vi "Read Plot Area Bounds.vi"(8 "error in (no error)":errorcluster, 11 "GraphChart.lvclass in":refnum<class "GraphChart.lvclass">) -> (0 "error out":errorcluster, 2 "Plot Bounds":T1, 3 "GraphChart.lvclass out":refnum<class "GraphChart.lvclass">)   [LabVIEW 2015, in "GraphChart.lvclass"]
uses:
  GraphChart.lvclass
  <vilib>/Utility/miscctls.llb/LVRectTypeDef.ctl
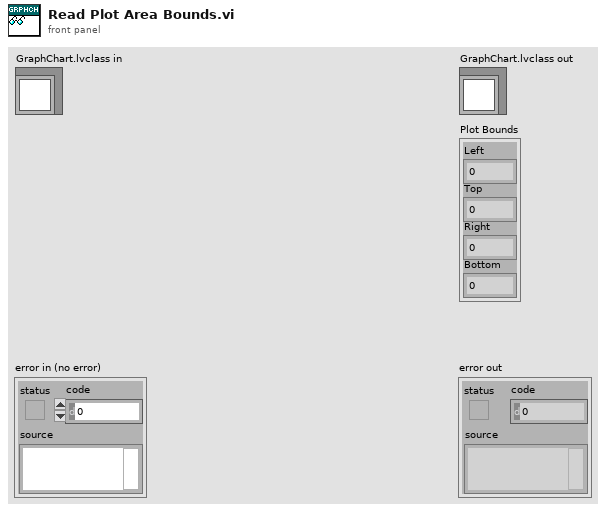
[diagram p1: front panel]
types:
  T1 = typedef "LVRectTypeDef.ctl" = cluster{"Left":i16, "Top":i16, "Right":i16, "Bottom":i16}
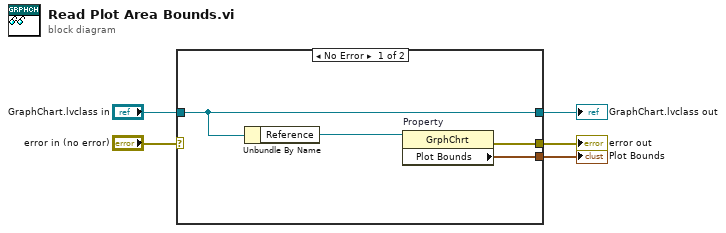
[diagram p0: block diagram]
diagram:
  n1 = case shown="No Error" "error in (no error)" {
    selector: "error in (no error)" -> [_ w11]
    tunnel: [w8 w11] -> w4
    tunnel: [w7 w10] -> w2
    tunnel: "GraphChart.lvclass in" -> [w7 w10]
    tunnel: [w9 _] -> w1
    frame No Error {
      n2 = Unbundle By Name(w7) -> ("Reference"=w6:refnum<vi>)
      n3 = property on="Property" class="GrphChrt"(reference=w6) -> (error out=w8:errorcluster, "Plot Bounds"=w9:T1)  [unwired: 1 in, 1 out]
    }
    frame Error {
    }
  }
  "error out" <- w4
  "GraphChart.lvclass out" <- w2
  "Plot Bounds" <- w1
